vi "Autonomous Independent.vi"() -> ()   [LabVIEW 2015]
doc: "This VI is called when autonomous begins, and will automatically be terminated when autonomous ends. You can carry out timed or sensor driven robot movement independently without needing to return to the caller."
uses:
  <vilib>/Rock Robotics/WPI/Utilities/WPI_GetSetVariantRefNum.vi
  <vilib>/Rock Robotics/Network Tables/NT Read String.vi
  <vilib>/Rock Robotics/Network Tables/NT Write Numeric Array.vi
  <vilib>/Rock Robotics/WPI/RobotDrive/WPI_RobotDriveArcadeDrive_Standard(NoSaturation).vi
panel:
  out "error out":errorcluster
  # "Be sure to right-click and choose Data Operations>>Make Current Value default if you want to save the array values with the VI"
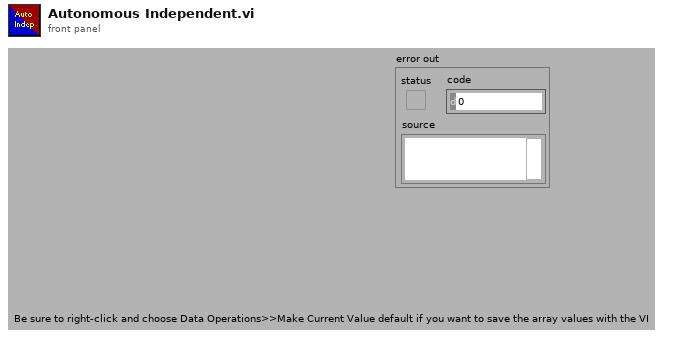
[diagram p1: front panel]
types:
  T1 = typedef "WPI_JoystickDevRef.ctl" = cluster{"Device":T2}
  T2 = typedef "WPI_JoystickDeviceEnum.ctl" = enum16{"USB 0", "USB 1", "USB 2", "USB 3", "USB 4", "USB 5"}
  T3 = typedef "WPI_MotorControlDeviceRef.ctl" = cluster{"DeviceStatus":errorcluster, "Type":T4, "PWM":cluster{"PWM Channel":T5, "DeadBand":T6}, "CAN":cluster{"Device Number":u8, "Control Mode":T7, "Semaphore":T8, "Max Vout":dbl, "TalonSRX Control Mode":T9}, "Invert":bool}
  T4 = typedef "WPI_MotorControlType.ctl" = enum16{"PWM", "CAN", "CANTalonSRX"}
  T5 = typedef "FPGA_DIOPWMChannel.ctl" = enum8{"PWM 0", "PWM 1", "PWM 2", "PWM 3", "PWM 4", "PWM 5", "PWM 6", "PWM 7", "PWM 8", "PWM 9", "PWM MXP 0", "PWM MXP 1", "PWM MXP 2", "PWM MXP 3", "PWM MXP 4", "PWM MXP 5", "PWM MXP 6", "PWM MXP 7", "PWM MXP 8", "PWM MXP 9", "Invalid"}
  T6 = typedef "WPI_PWMDeadband.ctl" = cluster{"Name":string, "maxPositivePwm":i32, "minPositivePwm":i32, "centerPwm":i32, "maxNegativePwm":i32, "minNegativePwm":i32, "angularRange":u16}
  T7 = typedef "WPI_CANJaguar_ControlMode.ctl" = enum8{"Percent VBus", "Current", "Speed", "Position", "Voltage"}
  T8 = typedef "Semaphore RefNum" = refnum<k1>
  T9 = typedef "WPI_CANTalonSRX_APIControlMode.ctl" = enum8{"Percent VBus", "Speed", "Position", "Slave", "Unchanged / Invalid", "Voltage Compensation", "Current", "Motion Profile"}
  T10 = typedef "WPI_RobotDriveDevRef.ctl" = cluster{"DevStatus":errorcluster, "Motors[]":T3[], "Square Inputs":bool, "Max Output":dbl}
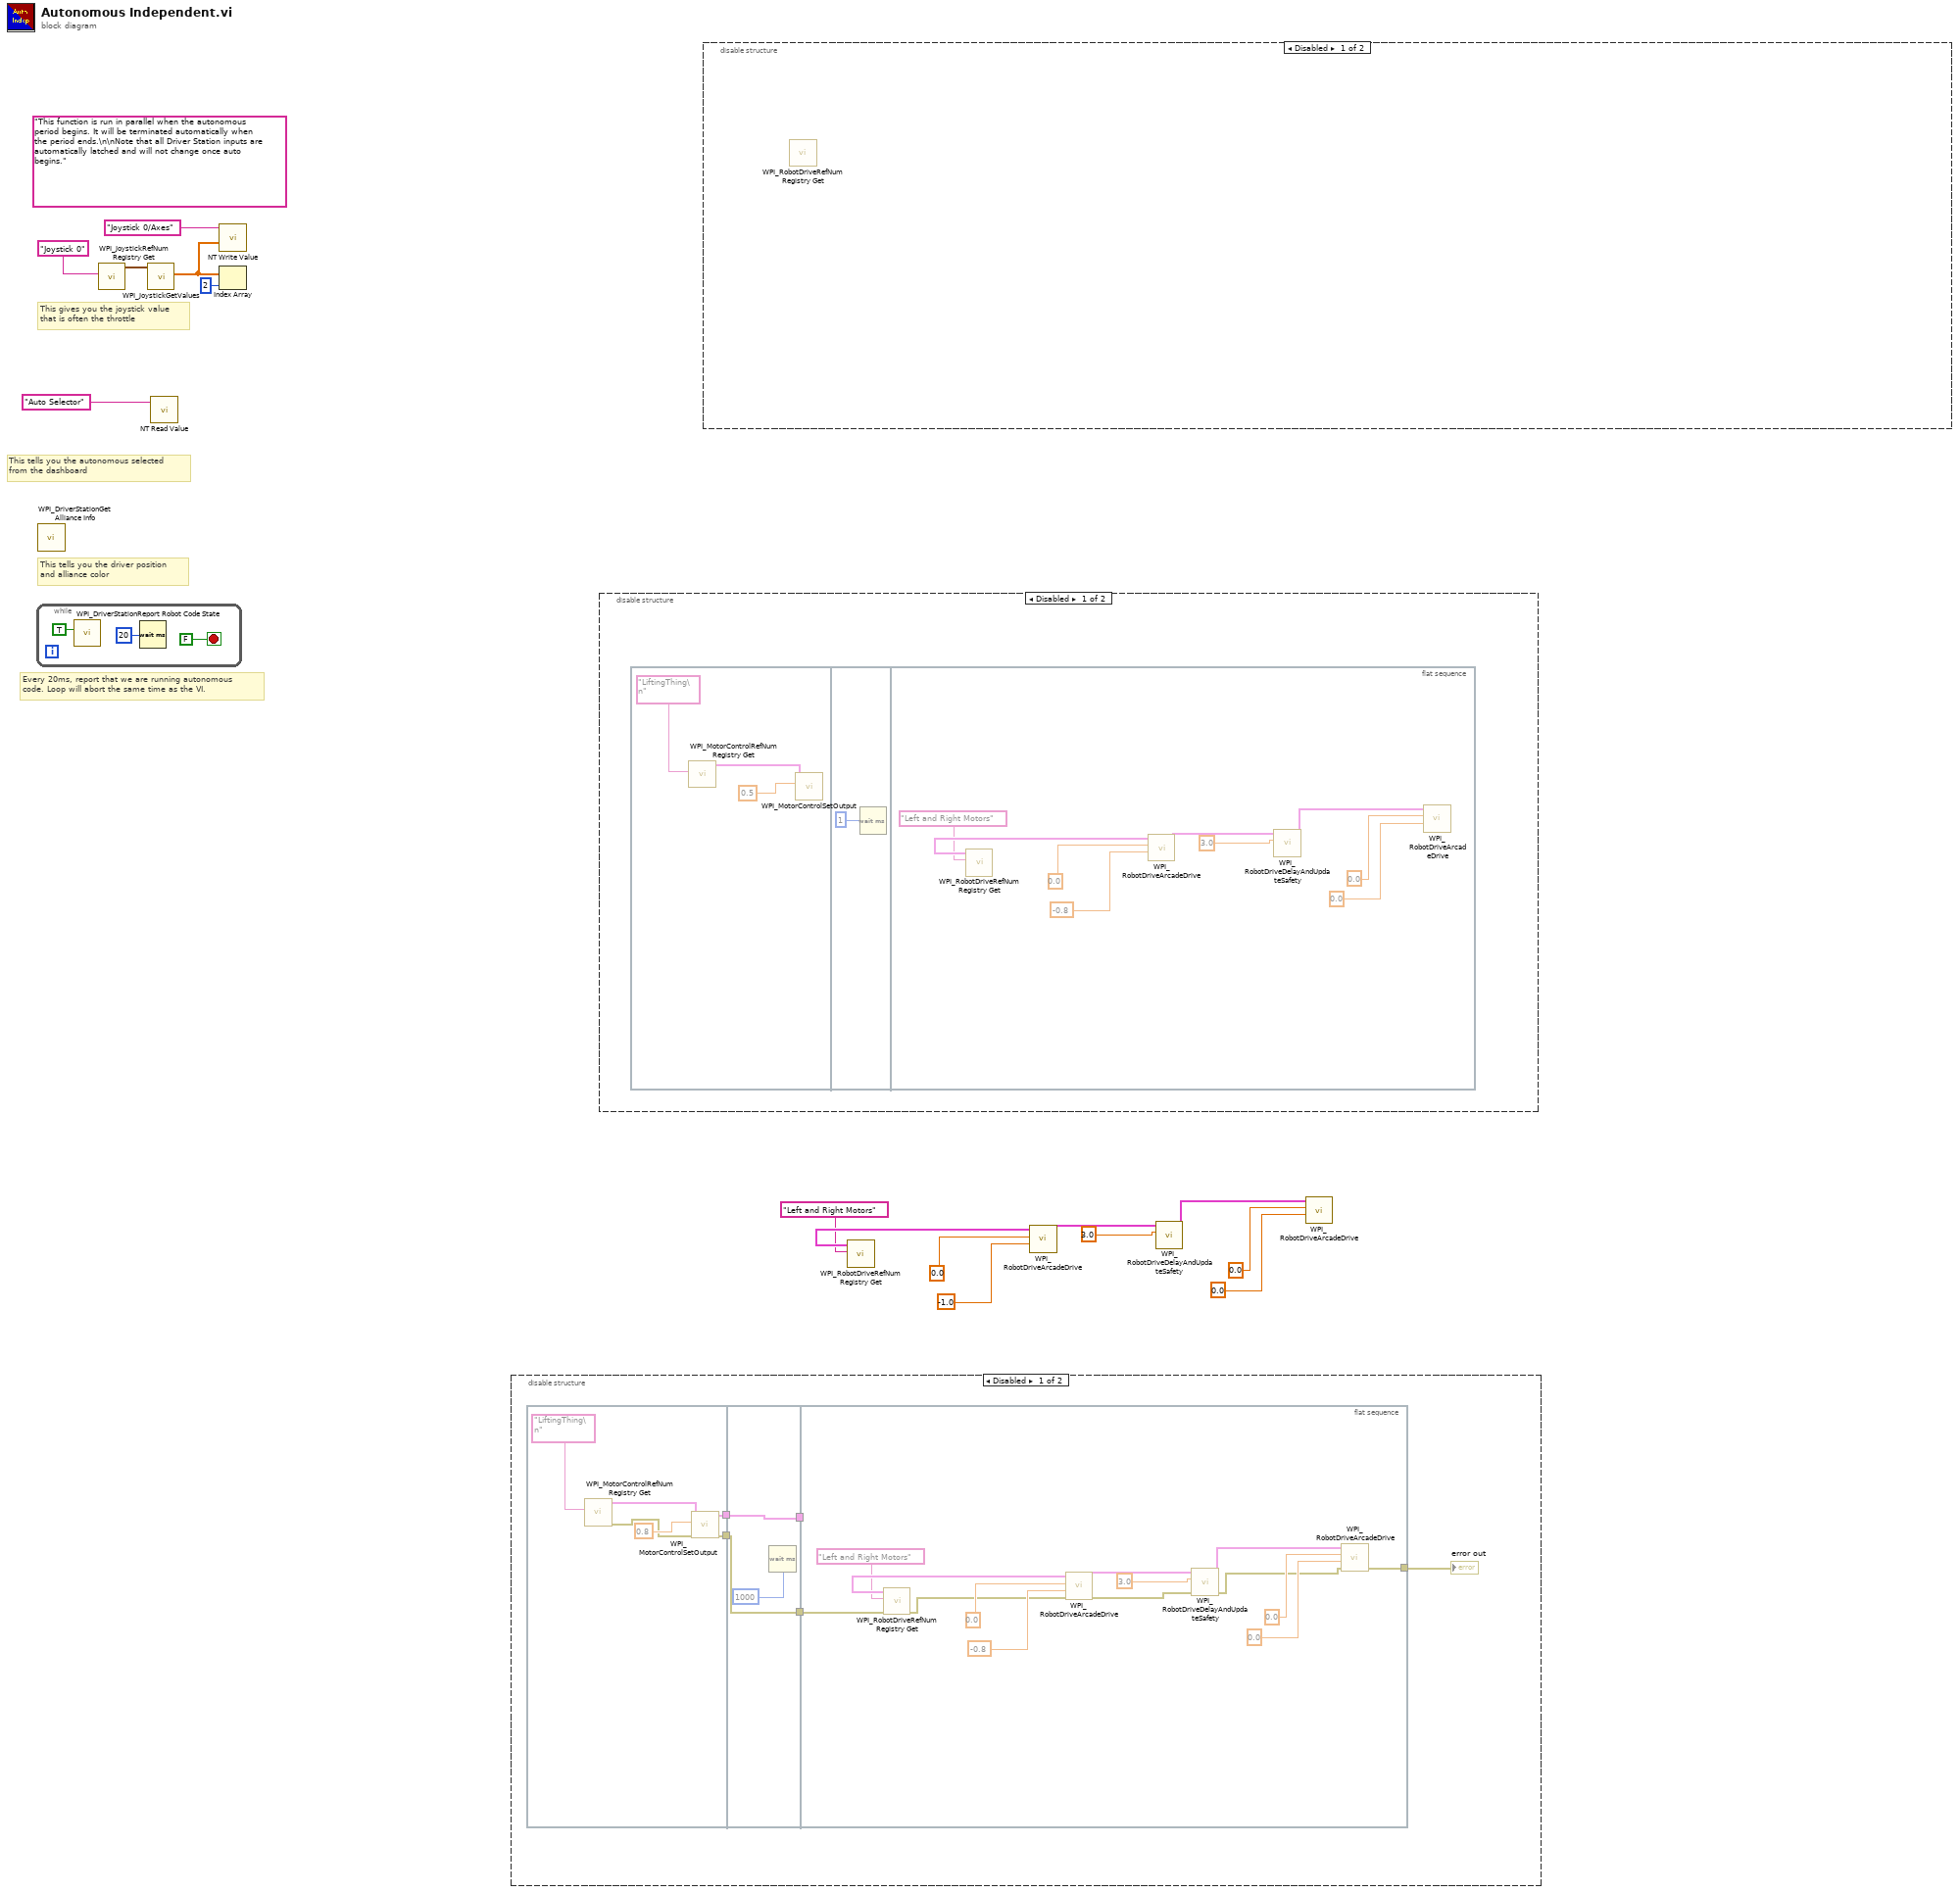
[diagram p0: block diagram]
diagram:
  (unwired) "This function is run in parallel when the autonomous period begins. It will be terminated automatically when the period ends.\n\nNote that all Driver Station inputs are automatically latched and will not change once auto begins."
  # "This tells you the autonomous selected\nfrom the dashboard"
  # "Every 20ms, report that we are running autonomous\ncode. Loop will abort the same time as the VI."
  # "This gives you the joystick value\nthat is often the throttle"
  # "This tells you the driver position\nand alliance color"
  n1 = while {
    stop <- FALSE stop-if-true
    n2 = call <vilib>:"WPI_DriverStationReport Robot Code State.vi"("Autonomous"=TRUE) -> ()  [unwired: 10 in, 1 out]
    n3 = Wait (ms)(milliseconds to wait=u32 20) -> ()  [unwired: 1 out]
  }
  n4 = call <vilib>:"WPI_DriverStationGet Alliance Info.vi"() -> ()  [unwired: 12 out]
  n5 = call <vilib>:"WPI_JoystickRefNum Registry Get.vi"("refnum name"="Joystick 0") -> ("JoystickDevRef"=w14:T1)  [unwired: 1 in, 9 out]
  n6 = call <vilib>:"WPI_JoystickGetValues.vi"("JoystickDevRef"=w14) -> ("Axes"=w11:dbl[])  [unwired: 6 in, 4 out]
  n7 = call-poly <vilib>:"NT Read Value.vi"("Name"="Auto Selector") -> ()  [unwired: 9 in, 2 out]
  n8 = call-poly <vilib>:"NT Write Value.vi"("Numeric Array"=w11, "Name"="Joystick 0/Axes") -> ()  [unwired: 9 in, 1 out]
  n9 = Index Array(array=w11, index=2) -> ()  [unwired: 1 out]
  n10 = disable-structure shown="Disabled" {
    frame Disabled {
      n11 = flat-sequence {
        tunnel: [w26] -> w23
        tunnel: [w25] -> w22
        tunnel: [w31] -> w21
        tunnel: w23 -> [w31]
        tunnel: [w30] -> w20
        tunnel: w22 -> [w30]
        tunnel: w21 -> [_]
        tunnel: w20 -> [w37]
        tunnel: [w33] -> w19
        frame #0 {
          n12 = call <vilib>:"WPI_MotorControlRefNum Registry Get.vi"("refnum name"="LiftingThing\n") -> ("error out"=w24:errorcluster, "MotorControlDevRef"=w28:T3)  [unwired: 9 in]
          n13 = call <vilib>:"WPI_MotorControlSetOutput.vi"("error in (no error)"=w24, "Output"=0.8 ("Motor Output"), "MotorControlDevRef"=w28) -> ("error out"=w25:errorcluster, "MotorControlDevRef"=w26:T3)  [unwired: 6 in, 1 out]
        }
        frame #1 {
          n14 = Wait (ms)(milliseconds to wait=u32 1000) -> ()  [unwired: 1 out]
        }
        frame #2 {
          n15 = call <vilib>:"WPI_RobotDriveRefNum Registry Get.vi"("error in (no error)"=w37, "refnum name"="Left and Right Motors") -> ("error out"=w36:errorcluster, "RobotDriveDevRef"=w43:T10)  [unwired: 8 out]
          n16 = call-poly <vilib>:"WPI_RobotDriveArcadeDrive.vi"("error in (no error)"=w36, "Y axis value"=-0.8, "X axis value"=0.0 ("Y axis value"), "RobotDriveDevRef"=w43) -> ("error out"=w35:errorcluster, "RobotDriveDevRef"=w44:T10)  [unwired: 5 in, 1 out]
          n17 = call <vilib>:"WPI_RobotDriveDelayAndUpdateSafety.vi"("error in (no error)"=w35, "Delay (s)"=3.0, "RobotDriveDevRef"=w44) -> ("error out"=w34:errorcluster, "RobotDriveDevRef 2"=w45:T10)  [unwired: 7 in]
          n18 = call-poly <vilib>:"WPI_RobotDriveArcadeDrive.vi"("error in (no error)"=w34, "Y axis value"=0.0, "X axis value"=0.0 ("Y axis value"), "RobotDriveDevRef"=w45) -> ("error out"=w33:errorcluster)  [unwired: 5 in, 2 out]
        }
      }
      "error out" <- w19
    }
    frame Enabled {
    }
  }
  n19 = disable-structure shown="Disabled" {
    frame Disabled {
      n20 = flat-sequence {
        frame #0 {
          n21 = call <vilib>:"WPI_MotorControlRefNum Registry Get.vi"("refnum name"="LiftingThing\n") -> ("MotorControlDevRef"=w48:T3)  [unwired: 9 in, 1 out]
          n22 = call <vilib>:"WPI_MotorControlSetOutput.vi"("Output"=0.5 ("Motor Output"), "MotorControlDevRef"=w48) -> ()  [unwired: 7 in, 3 out]
        }
        frame #1 {
          n23 = Wait (ms)(milliseconds to wait=u32 1) -> ()  [unwired: 1 out]
        }
        frame #2 {
          n24 = call <vilib>:"WPI_RobotDriveRefNum Registry Get.vi"("refnum name"="Left and Right Motors") -> ("RobotDriveDevRef"=w56:T10)  [unwired: 1 in, 9 out]
          n25 = call-poly <vilib>:"WPI_RobotDriveArcadeDrive.vi"("Y axis value"=-0.8, "X axis value"=0.0 ("Y axis value"), "RobotDriveDevRef"=w56) -> ("RobotDriveDevRef"=w57:T10)  [unwired: 6 in, 2 out]
          n26 = call <vilib>:"WPI_RobotDriveDelayAndUpdateSafety.vi"("Delay (s)"=3.0, "RobotDriveDevRef"=w57) -> ("RobotDriveDevRef 2"=w58:T10)  [unwired: 8 in, 1 out]
          n27 = call-poly <vilib>:"WPI_RobotDriveArcadeDrive.vi"("Y axis value"=0.0, "X axis value"=0.0 ("Y axis value"), "RobotDriveDevRef"=w58) -> ()  [unwired: 6 in, 3 out]
        }
      }
    }
    frame Enabled {
    }
  }
  n28 = disable-structure shown="Disabled" {
    frame Disabled {
      n29 = call <vilib>:"WPI_RobotDriveRefNum Registry Get.vi"() -> ("RobotDriveDevRef"=w60:T10, "refnum name"=w61:string)  [unwired: 1 in, 9 out]
    }
    frame Enabled {
    }
  }
  n30 = call <vilib>:"WPI_RobotDriveRefNum Registry Get.vi"("refnum name"="Left and Right Motors") -> ("RobotDriveDevRef"=w6:T10)  [unwired: 1 in, 9 out]
  n31 = call-poly <vilib>:"WPI_RobotDriveArcadeDrive.vi"("Y axis value"=-1.0, "X axis value"=0.0 ("Y axis value"), "RobotDriveDevRef"=w6) -> ("RobotDriveDevRef"=w7:T10)  [unwired: 6 in, 2 out]
  n32 = call <vilib>:"WPI_RobotDriveDelayAndUpdateSafety.vi"("Delay (s)"=3.0, "RobotDriveDevRef"=w7) -> ("RobotDriveDevRef 2"=w8:T10)  [unwired: 8 in, 1 out]
  n33 = call-poly <vilib>:"WPI_RobotDriveArcadeDrive.vi"("Y axis value"=0.0, "X axis value"=0.0 ("Y axis value"), "RobotDriveDevRef"=w8) -> ()  [unwired: 6 in, 3 out]
